vi "TCP Read - Discard Buffer.vi"(8 "error in":errorcluster, 11 "TCP Network Connection in":refnum<k5>) -> (0 "error out":errorcluster, 2 "Discarded Buffer Text":string, 3 "TCP Network Connection out":refnum<k5>)   [LabVIEW 2017, in "Communications Library.lvlib"]
doc: "Clears all characters from the received buffer and outputs them as a single string.\n\nIgnores timeout errors."
uses:
  Communications Library.lvlib
  Error 5102 - DTACQ unit replied with an error--const.vi
  <vilib>/Utility/error.llb/Error Cluster From Error Code.vi
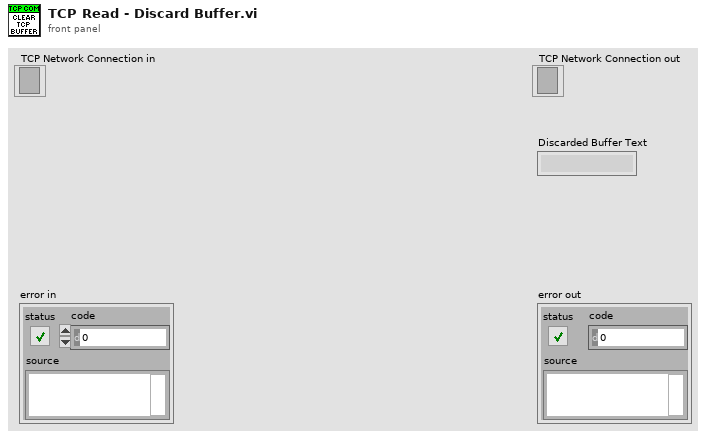
[diagram p1: front panel]
types:
  T1 = enum16{"Standard", "Buffered", "CRLF", "Immediate"}
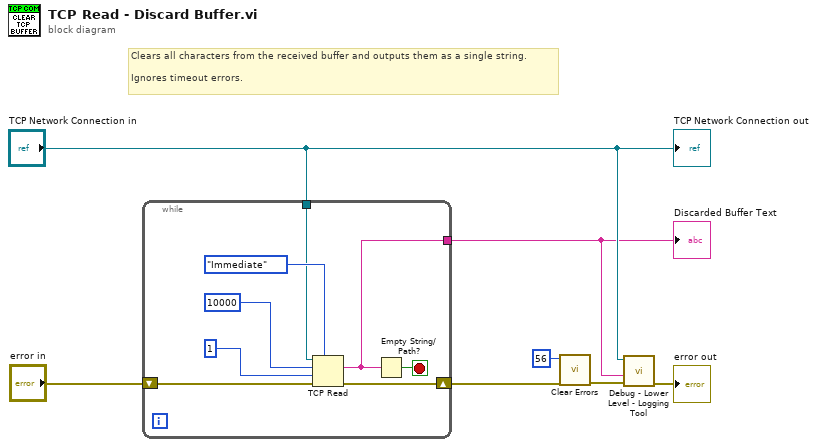
[diagram p0: block diagram]
diagram:
  # "Clears all characters from the received buffer and outputs them as a single string.\n\nIgnores timeout errors."
  n1 = while {
    tunnel: "TCP Network Connection in" -> [w12]
    shift-right: [w10] -> w6
    shift-left: "error in" -> [w15]
    tunnel: [w8] -> w1
    stop <- w9 stop-if-true
    n2 = TCP Read(connection ID=w12, bytes to read=10000, error in (no error)=w15, 7:T1."Immediate" ("mode (standard)"), 9:1 ("timeout ms (25000)")) -> (data out=w8:string, error out=w10:errorcluster)  [unwired: 1 out]
    n3 = Empty String/Path?(string/path=w8) -> (empty?=w9:bool)
  }
  "Discarded Buffer Text" <- w1
  n4 = call <vilib>:"Clear Errors.vi"("error in (no error)"=w6, "specific error code to clear (0: all)"=56) -> ("error out"=w4:errorcluster)  [unwired: 4 in, 1 out]
  n5 = call "Debug - Lower Level - Logging Tool.vi"("Error In"=w4, "Data Received"=w1, "TCP Network Connecion In"="TCP Network Connection in") -> ("Error Out"=→"error out":errorcluster)  [unwired: 7 in, 1 out]
  "TCP Network Connection out" <- "TCP Network Connection in"
